vi "Direction Finder.vi"(10 "Filtered Right Drive Rate":dbl, 11 "Filtered Left Drive Rate":dbl) -> (3 "Direction of travel":enum16{"Backward", "Forward", "Spin"}(ring))   [LabVIEW 2013]
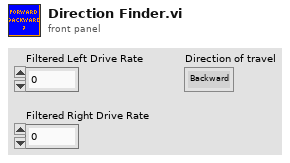
[diagram p1: front panel]
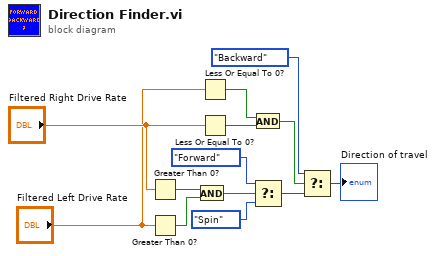
[diagram p0: block diagram]
diagram:
  n1 = Greater Than 0?(x="Filtered Right Drive Rate") -> (x > 0?=w2:bool)
  n2 = Greater Than 0?(x="Filtered Left Drive Rate") -> (x > 0?=w1:bool)
  n3 = And(x=w2, y=w1) -> (x .and. y?=w3:bool)
  n4 = Less Or Equal To 0?(x="Filtered Left Drive Rate") -> (x <= 0?=w6:bool)
  n5 = Less Or Equal To 0?(x="Filtered Right Drive Rate") -> (x <= 0?=w7:bool)
  n6 = And(x=w6, y=w7) -> (x .and. y?=w8:bool)
  n7 = Select(t=enum16{"Backward", "Forward", "Spin"}."Forward" ("Direction of travel"), s=w3, f=enum16{"Backward", "Forward", "Spin"}."Spin" ("Direction of travel")) -> (s? t:f=w12:enum16{"Backward", "Forward", "Spin"})
  n8 = Select(t=enum16{"Backward", "Forward", "Spin"}."Backward" ("Direction of travel"), s=w8, f=w12) -> (s? t:f=→"Direction of travel":enum16{"Backward", "Forward", "Spin"})
